vi "tsa_Single Side Spectrum.vi"(1 "FFT {X}":dbl[](array[numeric])) -> (0 "FFT {X}":dbl[](array[numeric]))   [LabVIEW 2020, in "NI_AALPro.lvlib"]
uses:
  <vilib>/Analysis/NI_AALPro.lvlib
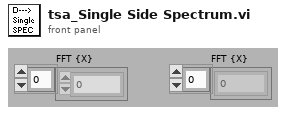
[diagram p1: front panel]
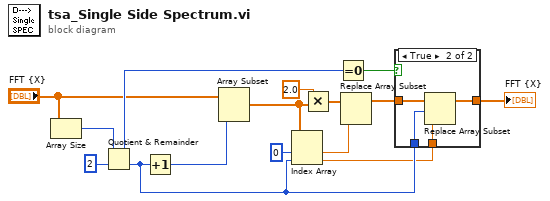
[diagram p0: block diagram]
diagram:
  n1 = Array Size(array="FFT {X}") -> (size(s)=w4:i32)
  n2 = Quotient & Remainder(x=w4, y=2) -> (x-y*floor(x/y)=w15:i32, floor(x/y)=w14:i32)
  n3 = Increment(x=w14) -> (x+1=w11:i32)
  n4 = Array Subset(array="FFT {X}", length=w11) -> (w3:dbl[])  [unwired: 1 in]
  n5 = Index Array(array=w3, index #1=0 ("index"), index #2=w14) -> (element #1=w9:dbl, element #2=w13:dbl)
  n6 = Multiply(x=2.0 ("y"), y=w3) -> (x*y=w8:dbl[])
  n7 = Equal To 0?(x=w15) -> (x = 0?=w10:bool)
  n8 = Replace Array Subset(array=w8, new element=w9) -> (w2:dbl[])  [unwired: 1 in]
  n9 = case shown="True" w10 {
    tunnel: w2 -> [w16 w20]
    tunnel: [w16 w19] -> w1
    tunnel: w14 -> [_ w18]
    tunnel: w13 -> [_ w17]
    frame False {
    }
    frame True {
      n10 = Replace Array Subset(array=w20, new element=w17, index=w18) -> (w19:dbl[])
    }
  }
  "FFT {X}" <- w1
